vi "MainUI.vi"() -> ()   [LabVIEW 2025]
panel:
  out "Error Out":errorcluster
  in  "Erro In":errorcluster
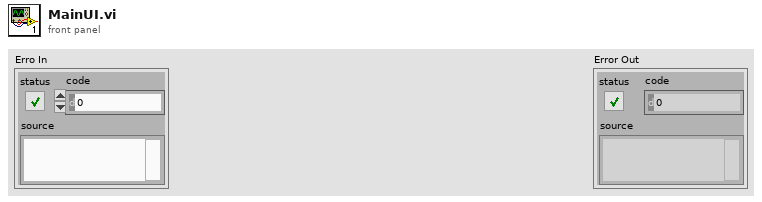
[diagram p1: front panel]
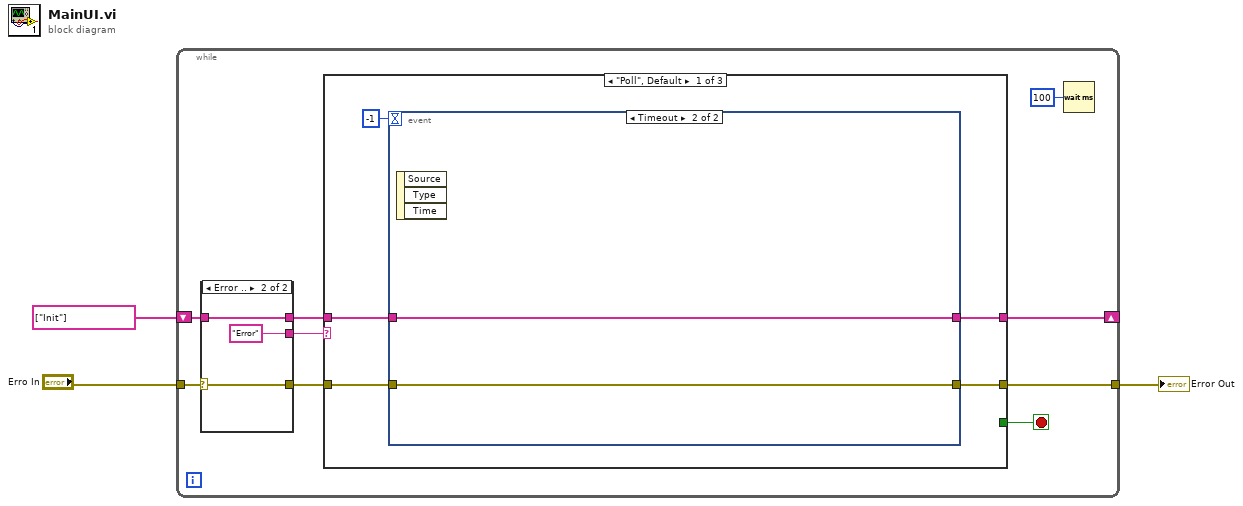
[diagram p0: block diagram]
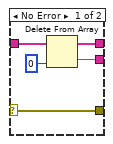
[diagram p2: hidden frame]
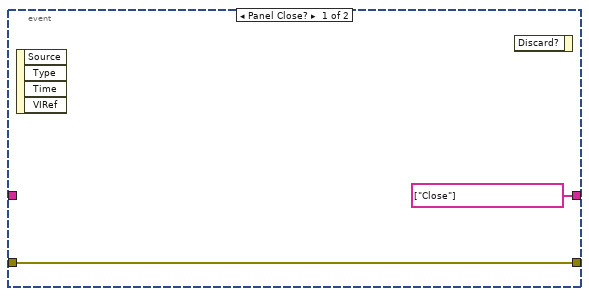
[diagram p3: hidden frame]
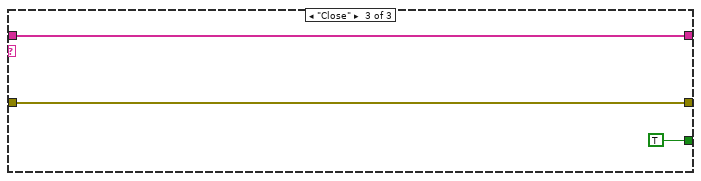
[diagram p5: hidden frame]
diagram:
  n1 = while {
    tunnel: [w11] -> w2
    tunnel: "Erro In" -> [w9]
    shift-right: [w6] -> _
    shift-left: string[] ["Init"] -> [w10]
    stop <- w4 stop-if-true
    n2 = case shown="Error .." w9 {
      selector: w9 -> [w16 w19]
      tunnel: w10 -> [w17 w20]
      tunnel: [w16 w19] -> w8
      tunnel: [w15 "Error" ("String")] -> w7
      tunnel: [w14 w20] -> w5
      frame No Error {
        n3 = Delete From Array(array=w17, index=0) -> (deleted portion=w15:string, array with subset deleted=w14:string[])  [unwired: 1 in]
      }
      frame Error {
      }
    }
    n4 = case shown="\"Poll\", Default" w7 {
      tunnel: [w24 w30 w34] -> w11
      tunnel: w8 -> [w23 w30 w34]
      tunnel: [w22 w31 w33] -> w6
      tunnel: w5 -> [w21 w31 w33]
      tunnel: [_ _ TRUE] -> w4
      frame "Poll", Default {
        n5 = event shown="[1] Timeout" {
          selector: _ -> [_ _]
          dyn-events: _ -> [_ _]
          timeout: -1 -> [_ _]
          tunnel: [w27 w29] -> w24
          tunnel: w23 -> [w27 w29]
          tunnel: [string[] ["Close"] w28] -> w22
          tunnel: w21 -> [_ w28]
          event Panel Close? {
            n6 = event-data() -> ()  [unwired: 1 in, 4 out]
            n7 = event-data() -> ()  [unwired: 2 in, 1 out]
          }
          event Timeout {
            n8 = event-data() -> ()  [unwired: 1 in, 3 out]
          }
        }
      }
      frame "Init" {
      }
      frame "Close" {
      }
    }
    n9 = Wait (ms)(milliseconds to wait=u32 100) -> ()  [unwired: 1 out]
  }
  "Error Out" <- w2
